vi "Get Autocal Current Step.vi"(0 "VISA Session In":refnum<visa-resource-name>="OXYMAT", 1 "Target Address":u8=16 format="%.0x", 2 "Source Address":u8=208 format="%.0x", 11 "error in (no error)":errorcluster) -> (4 "VISA Session Out":refnum<visa-resource-name>, 6 "Message Header":T2 {"Source Address" format="%.0x"; "Target Address" format="%.0x"}, 10 "Autocal Step":T1(ring), 13 "Success":bool, 15 "error out":errorcluster)   [LabVIEW 2020]
doc: "Using the Siemens ELAN protocol, getsthe current Autocal step (as an enumerated value) from the addressed analyzer. Also returns a boolean indicating that the addressed device provided a valid response.\n\n$Revision:: 0 $\n$Modtime:: yy-mm-dd hh:mm $\n$Author:: Dboyd $"
uses:
  Message Header.ctl
  Channel Status.ctl
  Siemens ELAN.lvlib
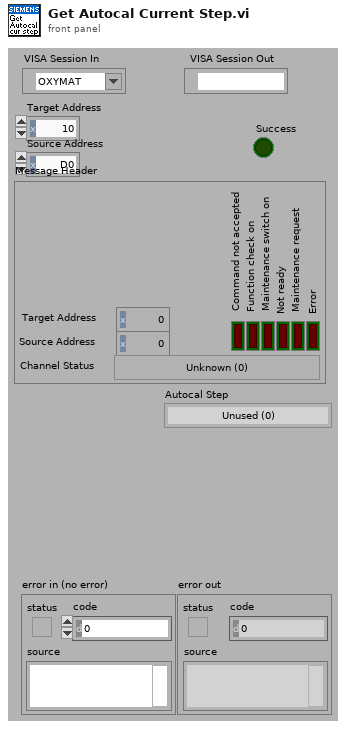
[diagram p1: front panel]
types:
  T1 = enum8{"Unused (0)", "Not Used", "Zero Gas 1", "Zero Gas 2", "Calibration Gas 1", "Calibration Gas 2", "Calibration Gas 3", "Calibration Gas 4", "Sample Gas Purging", "Intermediate Sample Gas Mode", "Signalling Contact", "Unused (>10)"}
  T2 = typedef "Siemens ELAN.lvlib/Message Header.ctl" = cluster{"Target Address":u8, "Source Address":u8, "Error":bool, "Maintenance request":bool, "Not ready":bool, "Maintenance switch on":bool, "Function check on":bool, "Command not accepted":bool, "Channel Status":T3}
  T3 = typedef "Siemens ELAN.lvlib/Channel Status.ctl" = enum8{"Unknown (0)", "Warm-up", "Pause", "Standby", "Measure", "Zero calibration", "Adjust component slope", "Unknown (7)", "Adjust curve dip", "Adjust linearization sensitivity", "Adjust temperature compensation", "Adjust pressure compensation", "Adjust linearization zero", "Adjust flow sensor", "Autocal", "Adjust phase", "Zero calibration of O2 sensor", "Synchronous zero calibration", "Purging for synchronous zero calibration", "Adjust analog output", "Adjust analog input", "Cleaning", "Unknown (>21)"}
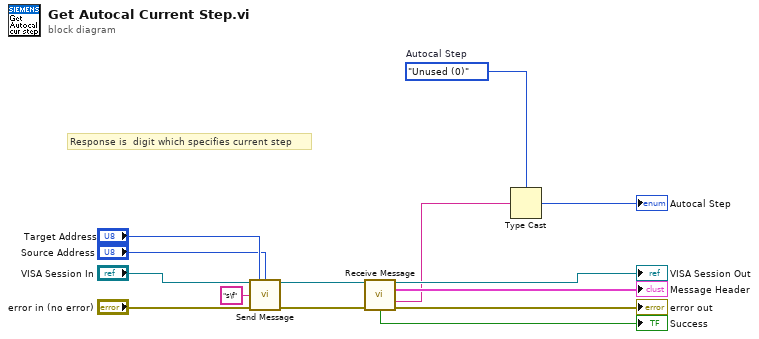
[diagram p0: block diagram]
diagram:
  w3 = T1."Unused (0)"  # Autocal Step
  # "Response is  digit which specifies current step"
  n1 = call "Send Message.vi"("VISA Session In"="VISA Session In", "Target Address"="Target Address", "Source Address"="Source Address", "Command"="s\f", "error in (no error)"="error in (no error)") -> ("VISA Session Out"=w14:refnum<visa-resource-name>, "error out"=w13:errorcluster)  [unwired: 8 in, 1 out]
  n2 = call "Receive Message.vi"("VISA Session In"=w14, "error in (no error)"=w13) -> ("VISA Session Out"=→"VISA Session Out":refnum<visa-resource-name>, "Message Header"=→"Message Header":T2, "Response"=w2:string, "Success"=→"Success":bool, "error out"=→"error out":errorcluster)  [unwired: 8 in, 1 out]
  n3 = Type Cast(type=w3, x=w2) -> (*(type *) &x=→"Autocal Step":T1)
